vi "Read SQL.vi"(8 "error in (no error)":errorcluster, 10 "SQL string":string, 11 "Data.PGQL in":refnum<class "LV-Data.PGSQL.lvclass">) -> (0 "error out":errorcluster, 1 "Result":string[][](array[string]), 2 "Trace":cluster{timestamp[], dbl[]}, 3 "Data.PGSQL out":refnum<class "LV-Data.PGSQL.lvclass">)   [LabVIEW 2019, in "LV-Data.PGSQL.lvclass"]
uses:
  LV-Data.PGSQL.lvclass
  LV-Data/Typedefs/Operation--enum.ctl
  LV-Data/LV-Data.lvclass
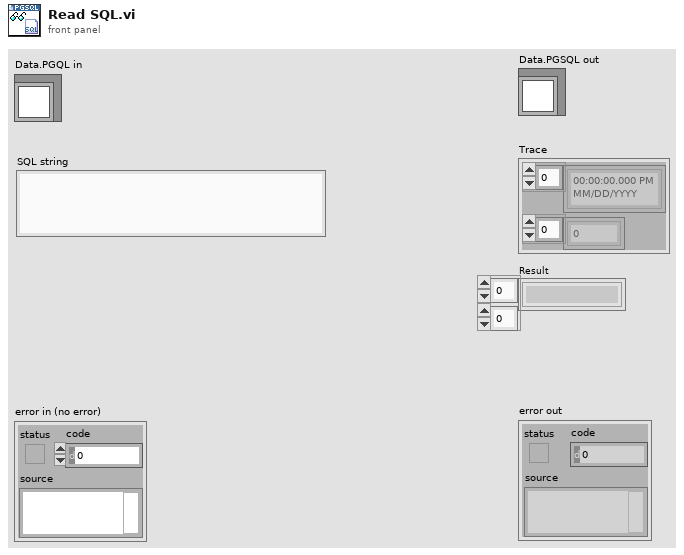
[diagram p1: front panel]
types:
  T1 = typedef "LV-Data.lvclass/Operation--enum.ctl" = enum16{"Read", "Write", "Write + Append"}
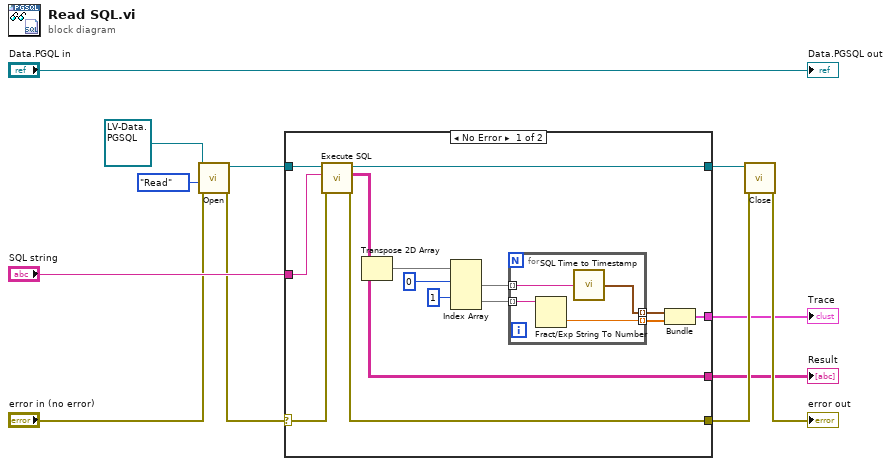
[diagram p0: block diagram]
diagram:
  n1 = call-dynamic "Open.vi"("error in (no error)"="error in (no error)", "Operation"=Operation--enum."Read", "Data.PG in"=refnum<class "LV-Data.PGSQL.lvclass"> refnum) -> ("error out"=w1:errorcluster, "Data.PG out"=w11:refnum<class "LV-Data.PGSQL.lvclass">)  [unwired: 7 in]
  n2 = case shown="No Error" w1 {
    selector: w1 -> [w22 w31]
    tunnel: w11 -> [w26 w32]
    tunnel: "SQL string" -> [w23 _]
    tunnel: [w25 w31] -> w9
    tunnel: [w24 w32] -> w10
    tunnel: [w14 _] -> w7
    tunnel: [w13 _] -> w6
    frame No Error {
      n3 = call "Execute SQL.vi"("error in"=w22, "SQL"=w23, "LV-Data.PGSQL"=w26) -> ("error out"=w25:errorcluster, "Result"=w13:string[][], "LV-Data.PGSQL out"=w24:refnum<class "LV-Data.PGSQL.lvclass">)  [unwired: 6 in]
      n4 = Transpose 2D Array(2D array=w13) -> (transposed array=w15:string[][])
      n5 = Index Array(array=w15, index (row) #1=0 ("index (row)"), index (row) #2=1 ("index (row)")) -> (element #1=w18:string[], element #2=w19:string[])  [unwired: 2 in]
      n6 = for {
        tunnel: w18 -> [w30] mode=indexing
        tunnel: w19 -> [w29] mode=indexing
        tunnel: [w28] -> w21 mode=indexing
        tunnel: [w27] -> w20 mode=indexing
        n7 = Fract/Exp String To Number(string=w29) -> (number=w28:dbl)  [unwired: 3 in, 1 out]
        n8 = call "SQL Time to Timestamp.vi"("Get:Get String"=w30) -> ("Time Stamp"=w27:timestamp)
      }
      n9 = Bundle(w20, w21) -> (w14:cluster{timestamp[], dbl[]})  [unwired: 1 in]
    }
    frame Error {
    }
  }
  "Trace" <- w7
  "Result" <- w6
  n10 = call-dynamic "Close.vi"("error in (no error)"=w9, "Data.PG in"=w10) -> ("error out"=→"error out":errorcluster)  [unwired: 8 in, 1 out]
  "Data.PGSQL out" <- "Data.PGQL in"
